vi "字符串移位显示.vi"(8 "错误输入":errorcluster, 10 "字符框大小":i32=36, 11 "字符串输入":string="仪器校准中!") -> (0 "错误输出":errorcluster, 3 "移位后字符串":string)   [LabVIEW 2016, in "数据传输系统.lvlib"]
panel:
  out "补位字符串":string
  out "数值":i32
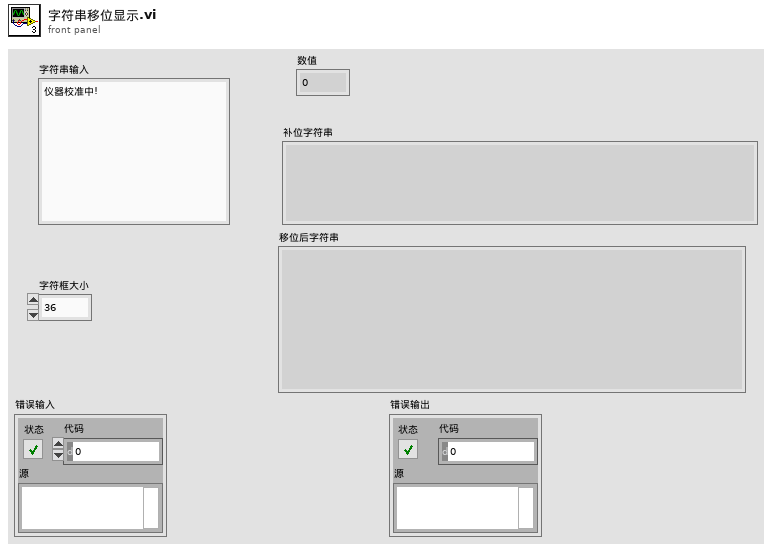
[diagram p1: front panel]
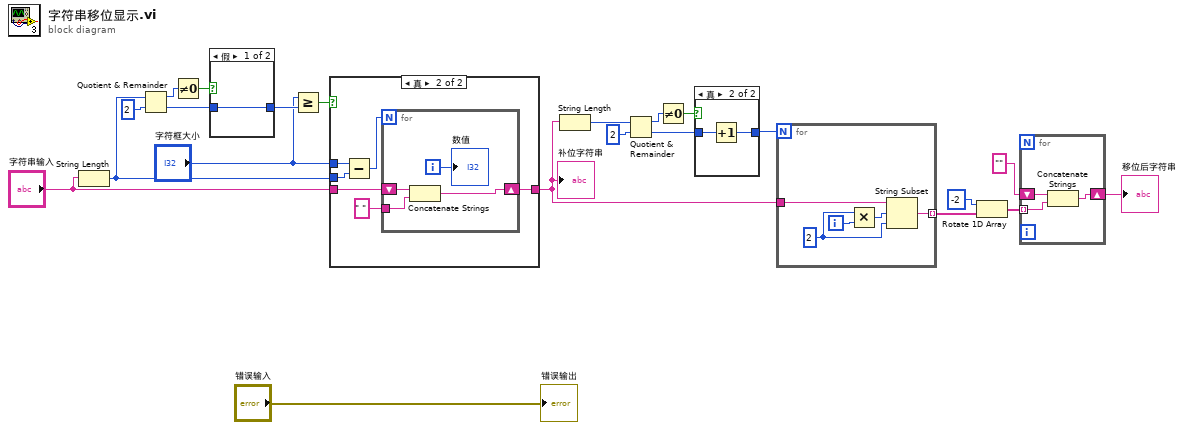
[diagram p0: block diagram]
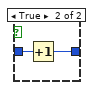
[diagram p3: hidden frame]
diagram:
  n1 = String Length(string="字符串输入") -> (length=w9:i32)
  n2 = Quotient & Remainder(x=w9, y=2) -> (x-y*floor(x/y)=w15:i32, floor(x/y)=w13:i32)
  n3 = Not Equal To 0?(x=w15) -> (x != 0?=w14:bool)
  n4 = case shown="假" w14 {
    tunnel: w13 -> [w23 w25]
    tunnel: [w23 w24] -> w11
    frame False {
    }
    frame True {
      n5 = Increment(x=w25) -> (x+1=w24:i32)
    }
  }
  n6 = Greater Or Equal?(x="字符框大小", y=w11) -> (x >= y?=w12:bool)
  n7 = case shown="真" w12 {
    tunnel: "字符框大小" -> [_ w32]
    tunnel: w9 -> [_ w31]
    tunnel: "字符串输入" -> [w26 w28]
    tunnel: [w26 w27] -> w10
    frame False {
    }
    frame True {
      n8 = Subtract(x=w32, y=w31) -> (x-y=w30:i32)
      n9 = for {
        N: w30 -> [_]
        tunnel: " " ("字符串") -> [w36]
        shift-right: [w35] -> w27
        shift-left: w28 -> [w34]
        i -> [w33]
        n10 = Concatenate Strings(w34, w36) -> (w35:string)
        "数值" <- w33
      }
    }
  }
  "补位字符串" <- w10
  n11 = String Length(string=w10) -> (length=w22:i32)
  n12 = Quotient & Remainder(x=w22, y=2) -> (x-y*floor(x/y)=w20:i32, floor(x/y)=w18:i32)
  n13 = Not Equal To 0?(x=w20) -> (x != 0?=w19:bool)
  n14 = case shown="真" w19 {
    tunnel: w18 -> [w37 w39]
    tunnel: [w37 w38] -> w17
    frame False {
    }
    frame True {
      n15 = Increment(x=w39) -> (x+1=w38:i32)
    }
  }
  n16 = for {
    N: w17 -> [_]
    tunnel: w10 -> [w43]
    tunnel: [w44] -> w8 mode=indexing
    i -> [w42]
    w41 = 2 ("长度（剩余）")
    n17 = Multiply(x=w41, y=w42) -> (x*y=w40:i32)
    n18 = String Subset(string=w43, offset (0)=w40, length (rest)=w41) -> (substring=w44:string)
  }
  n19 = Rotate 1D Array(1:w8, 2:-2 ("n")) -> (0:w6:string[])
  n20 = for {
    tunnel: w6 -> [w47] mode=indexing
    shift-right: [w45] -> w1
    shift-left: "" -> [w46]
    n21 = Concatenate Strings(w46, w47) -> (w45:string)
  }
  "移位后字符串" <- w1
  "错误输出" <- "错误输入"
